vi "OvernightTemp.vi"() -> ()   [LabVIEW 2013]
panel:
  in  "error in (no error)":errorcluster
  out "Sweep":i16
  out "Array":dbl[](array[numeric])
  in  "Step (K)":dbl=10.0 min=-4.0 max=4.0 step=1.0 format="%#.3g"
  in  "Start sweeping":bool
  in  "Final T (K)":dbl=200.0 min=-4.0 max=4.0 step=0.1 format="%.3f"
  in  "Initial T (K)":dbl=10.0 min=-4.0 max=4.0 step=0.1 format="%.4f"
  # "Define interval of gate voltage\nfor main Keithley 2400 (address 12):"
  # "Settemperatures at which sweeps\nare made:"
  # "SourceMeter (address 13)"
  # "min."
  # "= approx."
  # "hours"
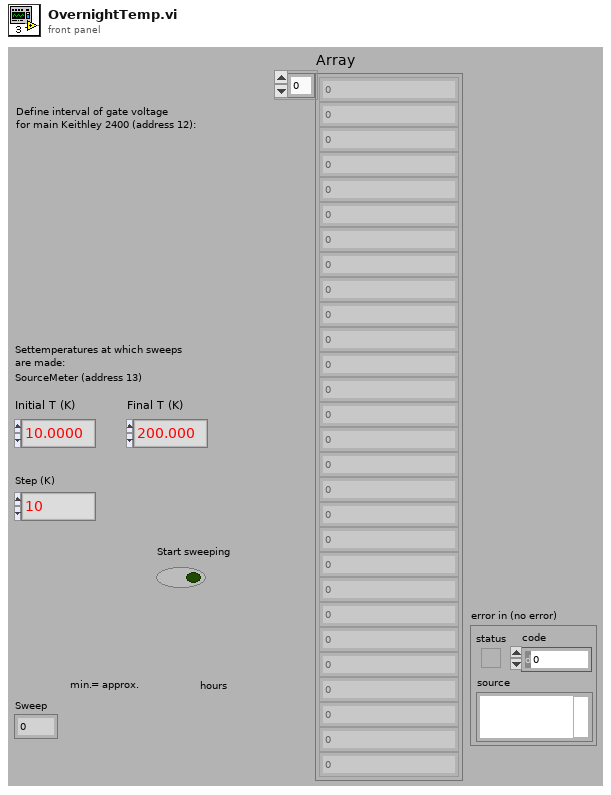
[diagram p1: front panel]
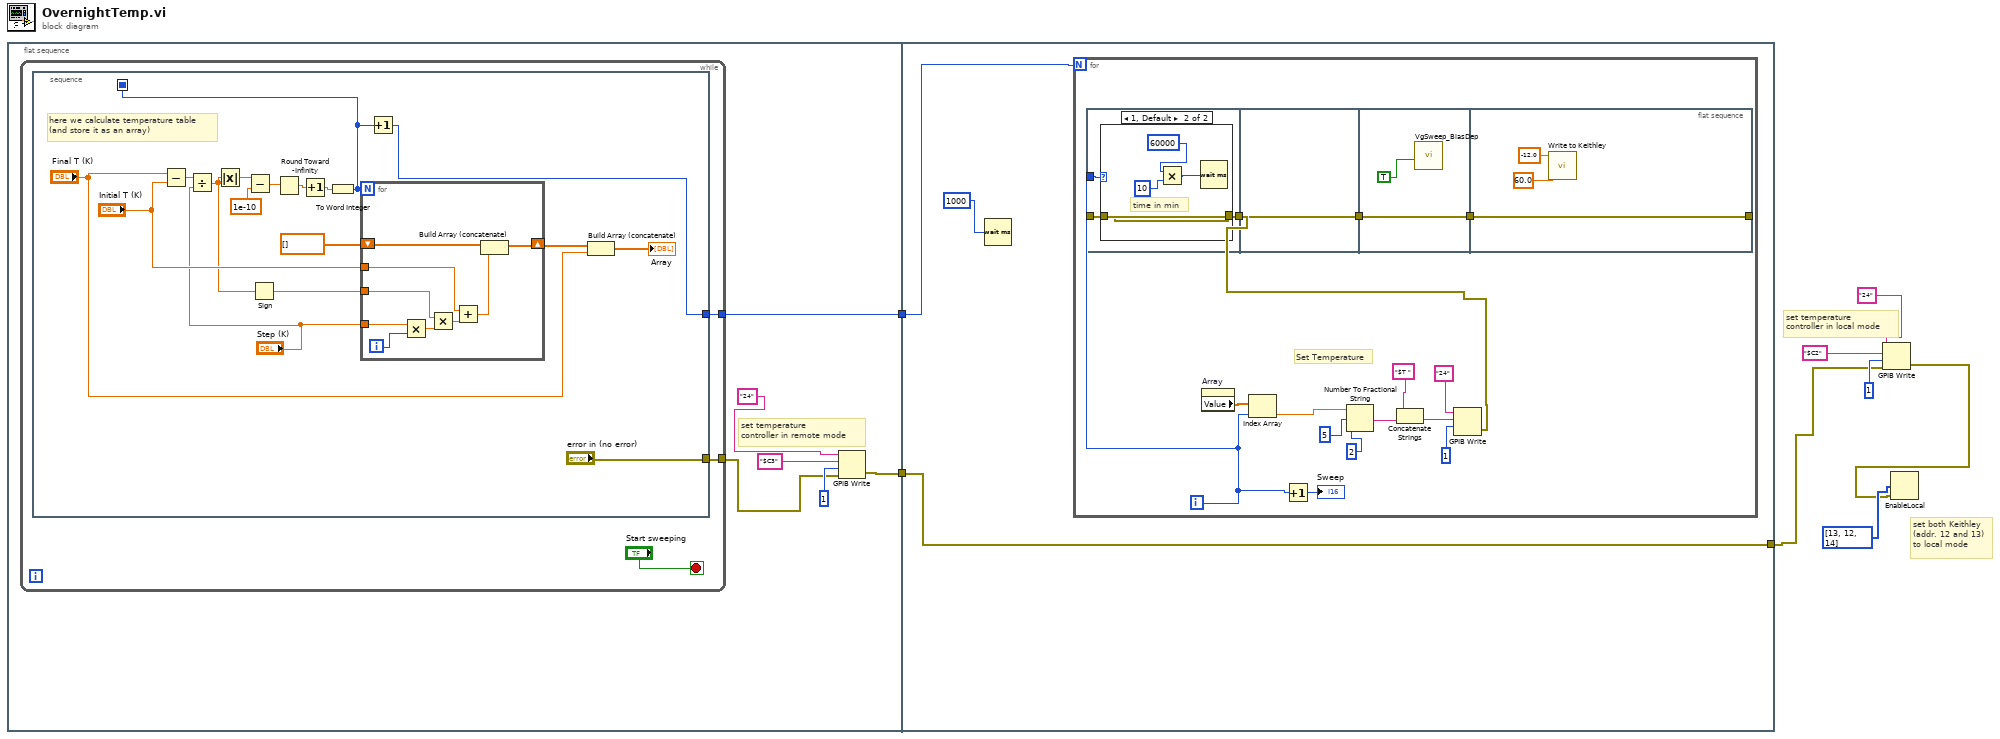
[diagram p0: block diagram]
diagram:
  # "set temperature\ncontroller in local mode"
  # "set both Keithley\n(addr. 12 and 13)\nto local mode"
  n1 = flat-sequence {
    tunnel: [w14] -> w8
    tunnel: [w11] -> w6
    tunnel: w8 -> [w46]
    tunnel: w6 -> [w45]
    tunnel: [w45] -> w2
    frame #0 {
      # "set temperature\ncontroller in remote mode"
      n2 = while {
        tunnel: [w16] -> w14
        tunnel: [w15] -> w10
        stop <- "Start sweeping" stop-if-true
        n3 = stacked-sequence {
          seq-local: [w20] -> [_]
          tunnel: [w19] -> w16
          tunnel: ["error in (no error)"] -> w15
          frame #0 {
            # "here we calculate temperature table\n(and store it as an array)"
            n4 = Subtract(x="Final T (K)", y="Initial T (K)") -> (x-y=w24:dbl)
            n5 = Divide(x=w24, y="Step (K)") -> (x/y=w23:dbl)
            n6 = Absolute Value(x=w23) -> (abs(x)=w33:dbl)
            n7 = Subtract(x=w33, y=1e-10) -> (x-y=w31:dbl)
            n8 = Sign(1:w23) -> (0:w30:dbl)
            n9 = Round Toward -Infinity(1:w31) -> (0:w25:dbl)
            n10 = Increment(x=w25) -> (x+1=w21:dbl)
            n11 = To Word Integer(number=w21) -> (16bit integer=w20:i16)
            n12 = for {
              N: w20 -> [_]
              shift-right: [w35] -> w28
              shift-left: dbl[] [] -> [w43]
              tunnel: "Step (K)" -> [w41]
              tunnel: w30 -> [w39]
              tunnel: "Initial T (K)" -> [w37]
              i -> [w40]
              n13 = Multiply(x=w41, y=w40) -> (x*y=w42:dbl)
              n14 = Multiply(x=w39, y=w42) -> (x*y=w38:dbl)
              n15 = Add(x=w37, y=w38) -> (x+y=w36:dbl)
              n16 = Build Array (concatenate)(w43, w36) -> (w35:dbl[])
            }
            n17 = Increment(x=w20) -> (x+1=w19:i16)
            n18 = Build Array (concatenate)(w28, "Final T (K)") -> (→"Array":dbl[])
          }
        }
      }
      n19 = GPIB Write(0:"24", 1:"$C3", 2:1, 3:w10) -> (6:w11:errorcluster)  [unwired: 1 in, 1 out]
    }
    frame #1 {
      n20 = Wait (ms)(milliseconds to wait=1000) -> ()  [unwired: 1 out]
      n21 = for {
        N: w46 -> [_]
        i -> [w47]
        # "Set Temperature"
        n22 = flat-sequence {
          tunnel: w51 -> [w63]
          tunnel: [w62] -> w48
          tunnel: w47 -> [w64]
          tunnel: [w70] -> w50
          tunnel: w48 -> [w70]
          tunnel: w50 -> [w72]
          tunnel: [w72] -> w49
          tunnel: w49 -> [w75]
          tunnel: [w75] -> _
          frame #0 {
            n23 = case shown="1, Default" w64 {
              tunnel: w63 -> [w65 w66]
              tunnel: [w65 w66] -> w62
              frame 0 {
              }
              frame 1, Default {
                # "time in min"
                n24 = Multiply(x=60000, y=10) -> (x*y=w68:i32)
                n25 = Wait (ms)(milliseconds to wait=w68) -> ()  [unwired: 1 out]
              }
            }
          }
          frame #1 {
          }
          frame #2 {
            n26 = call "VgSweep_BiasDep.vi"("Start sweeping"=TRUE) -> ()  [unwired: 11 in]
          }
          frame #3 {
            n27 = call "Write to Keithley.vi"("Number of Points"=60.0, "Target Value"=-12.0) -> ()  [unwired: 10 in]
          }
        }
        n28 = property on="Array" class="Arr (strict)"() -> ("Value"=w61:dbl[])  [unwired: 2 in, 2 out]
        n29 = Index Array(array=w61, index=w47) -> (element=w52:dbl)
        n30 = Increment(x=w47) -> (x+1=→"Sweep":i32)
        n31 = Number To Fractional String(number=w52, width (-)=5, precision (6)=2) -> (F-format string=w57:string)  [unwired: 1 in]
        n32 = Concatenate Strings("$T ", w57) -> (w56:string)
        n33 = GPIB Write(0:"24", 1:w56, 2:1) -> (6:w51:errorcluster)  [unwired: 2 in, 1 out]
      }
    }
  }
  n34 = GPIB Write(0:"24", 1:"$C2", 2:1, 3:w2) -> (6:w1:errorcluster)  [unwired: 1 in, 1 out]
  n35 = EnableLocal(2:w1, 3:i32[] [13, 12, 14]) -> ()  [unwired: 1 in, 2 out]
